vi "Exit Timer.vi"(8 "error in (no error)":errorcluster, 11 "Timer Handler":T1) -> (0 "error out":errorcluster)   [LabVIEW 2024]
doc: "Exits the timer by generating exit timer events."
uses:
  Timer Handler.ctl
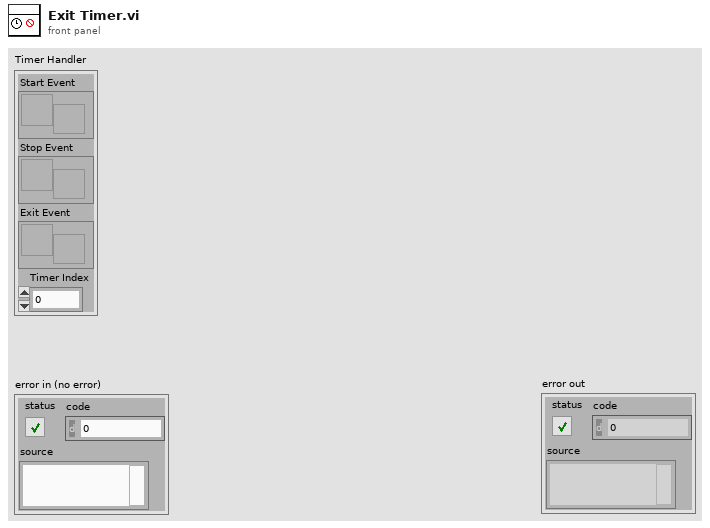
[diagram p1: front panel]
types:
  T1 = typedef "Timer Handler.ctl" = cluster{"Start Event":refnum<user-event>, "Stop Event":refnum<user-event>, "Exit Event":refnum<user-event>, "Timer Index":u32}
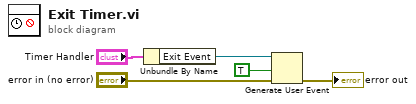
[diagram p0: block diagram]
diagram:
  n1 = Unbundle By Name("Timer Handler") -> ("Exit Event"=w1:refnum<user-event>)
  n2 = Generate User Event(user event=w1, event data cluster=TRUE ("event data"), error in="error in (no error)") -> (error out=→"error out":errorcluster)  [unwired: 1 in, 1 out]
